vi "init_station_keeping.vi"(6 "Buoy SE":T1 {"North" format="%#_10f"; "East" format="%#_8f"}, 7 "Buoy NE":T1 {"North" format="%#_10f"; "East" format="%#_8f"}, 8 "Buoy SW":T1 {"North" format="%#_10f"; "East" format="%#_8f"}, 11 "Buoy NW":T1 {"North" format="%#_10f"; "East" format="%#_8f"}) -> (3 "Mission out":refnum<class "Mission.lvclass">)   [LabVIEW 2011, in "Mission.lvclass"]
uses:
  Mission.lvclass
  2 Typedefs/UTM Location.ctl
  Mission.lvclass/Mission.ctl
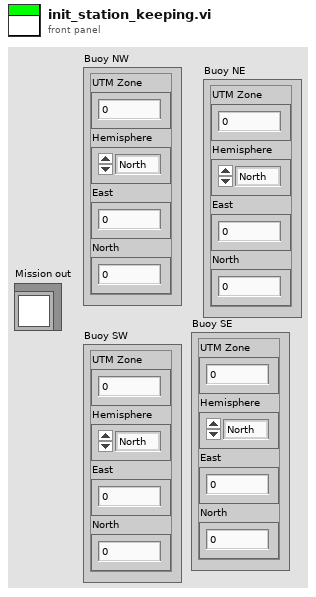
[diagram p1: front panel]
types:
  T1 = typedef "UTM Location.ctl" = cluster{"UTM Zone":dbl, "Hemisphere":enum16{"North", "South"}, "East":dbl, "North":dbl}
  T2 = enum16{"Round Buoy", "Drive", "Pass Buoys", "Station Keeping"}
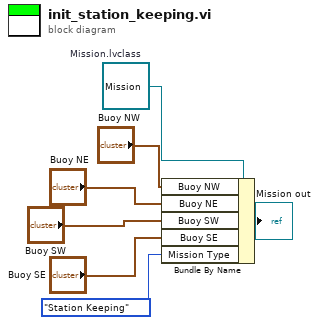
[diagram p0: block diagram]
diagram:
  w7 = refnum<class "Mission.lvclass"> refnum  # Mission.lvclass
  n1 = Bundle By Name(cluster=w7, "Buoy NW"="Buoy NW", "Buoy NE"="Buoy NE", "Buoy SW"="Buoy SW", "Buoy SE"="Buoy SE", "Mission Type"=T2."Station Keeping") -> (→"Mission out":refnum<class "Mission.lvclass">)
